vi "Set from JSON string.vi"(8 "error in (no error)":errorcluster, 10 "JSON stream":string, 11 "JSON Value in":refnum<class "JSON Value.lvclass">) -> (0 "error out":errorcluster, 2 "rest of JSON stream":string, 3 "JSON Value out":refnum<class "JSON Value.lvclass">)   [LabVIEW 2011, in "JSON Value.lvclass"]
doc: "Converts a <b>JSON stream</b> into a <b>JSON Value</b>.\n\nCopyright 2012 James David Powell, Shaun Rumbell and Ton Plomp\nMore information on http://lavag.org/topic/16217-cr-json-labview"
uses:
  JSON Value.lvclass
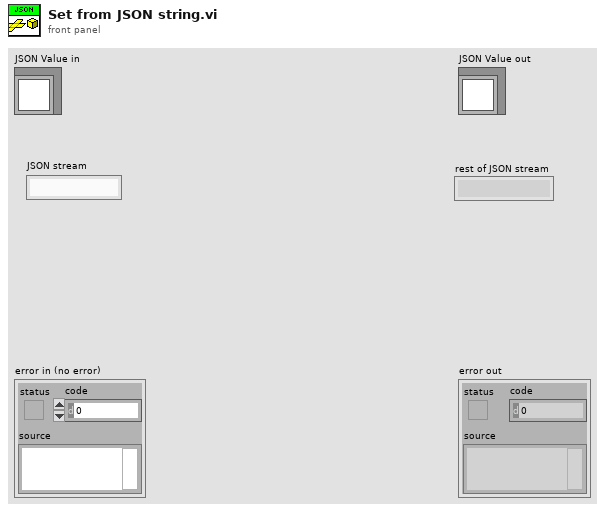
[diagram p1: front panel]
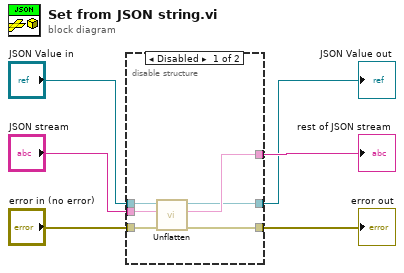
[diagram p0: block diagram]
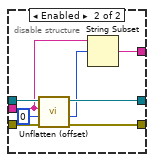
[diagram p2: hidden frame]
diagram:
  n1 = disable-structure shown="Disabled" {
    disable-tunnel: "JSON Value in" -> [w12 w20]
    disable-tunnel: "JSON stream" -> [w11 w15]
    disable-tunnel: "error in (no error)" -> [w10 w19]
    disable-tunnel: [w9 w18] -> w3
    disable-tunnel: [w8 w13] -> w2
    disable-tunnel: [w7 w17] -> w1
    frame Disabled {
      n2 = call-dynamic "Unflatten.vi"("error in (no error)"=w10, "JSON stream"=w11, "JSON Value in"=w12) -> ("error out"=w9:errorcluster, "rest of JSON stream"=w8:string, "JSON Value out"=w7:refnum<class "JSON Value.lvclass">)  [unwired: 5 in, 1 out]
    }
    frame Enabled {
      n3 = call-dynamic "Unflatten (offset).vi"("error in (no error)"=w19, "offset (0)"=0, "JSON stream"=w15, "JSON Value in"=w20) -> ("error out"=w18:errorcluster, "offset"=w14:i32, "JSON Value out"=w17:refnum<class "JSON Value.lvclass">)  [unwired: 4 in, 1 out]
      n4 = String Subset(string=w15, offset (0)=w14) -> (substring=w13:string)  [unwired: 1 in]
    }
  }
  "error out" <- w3
  "JSON Value out" <- w1
  "rest of JSON stream" <- w2
